vi "Server Single Connection.vi"() -> ()   [LabVIEW 2013]
doc: "This WebSockets API example VI acts as a server for an incoming websockets connection. Receives/sends string data to the connected client."
uses:
  WebSockets/WebSocket Server/WebSocket Server.lvclass
  WebSockets/WebSocket/WebSocket.lvclass/WebSocket.ctl
  WebSockets/WebSocket Server/WebSocket Server.lvclass/WebSocket Server.ctl
  WebSockets/WebSocket/Read Return Headers.vi
  WebSockets/WebSocket Server/Read Request URI.vi
  Sockets/VISA TCP Socket/VISA TCP.lvclass
panel:
  out "Request URI":string
  out "HTTP Headers":variant
  in  "Stop":bool
  out "Received Data":string
  in  "Send":bool
  in  "Data":string
  # "WebSockets Server Example"
  # "This VI is a simple example of sending/receiving data using WebSockets.\nIt waits for a single incoming WebSockets connection on Port 6123 and\nthen displays incoming string data. Strings can also be sent back to the client.\n\nInstructions for use:\n1) Run this VI\n2) Open the index.html file located in the examples folder or the 'Client Single Connection' example\n3) The index.html will display the status of the connection and once established, data can be sent/received from either this VI or the index.html file."
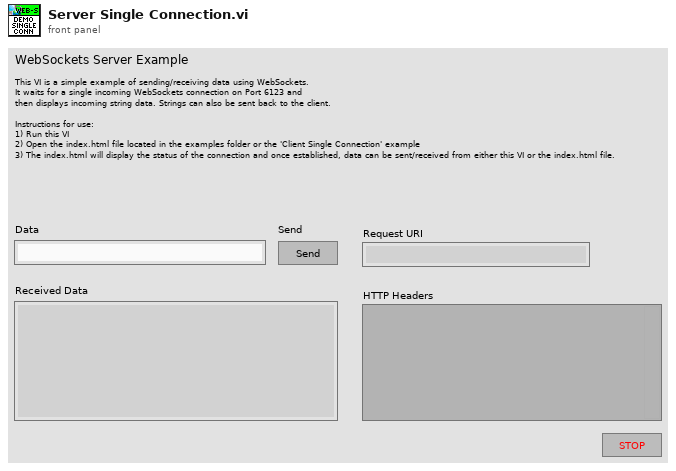
[diagram p1: front panel]
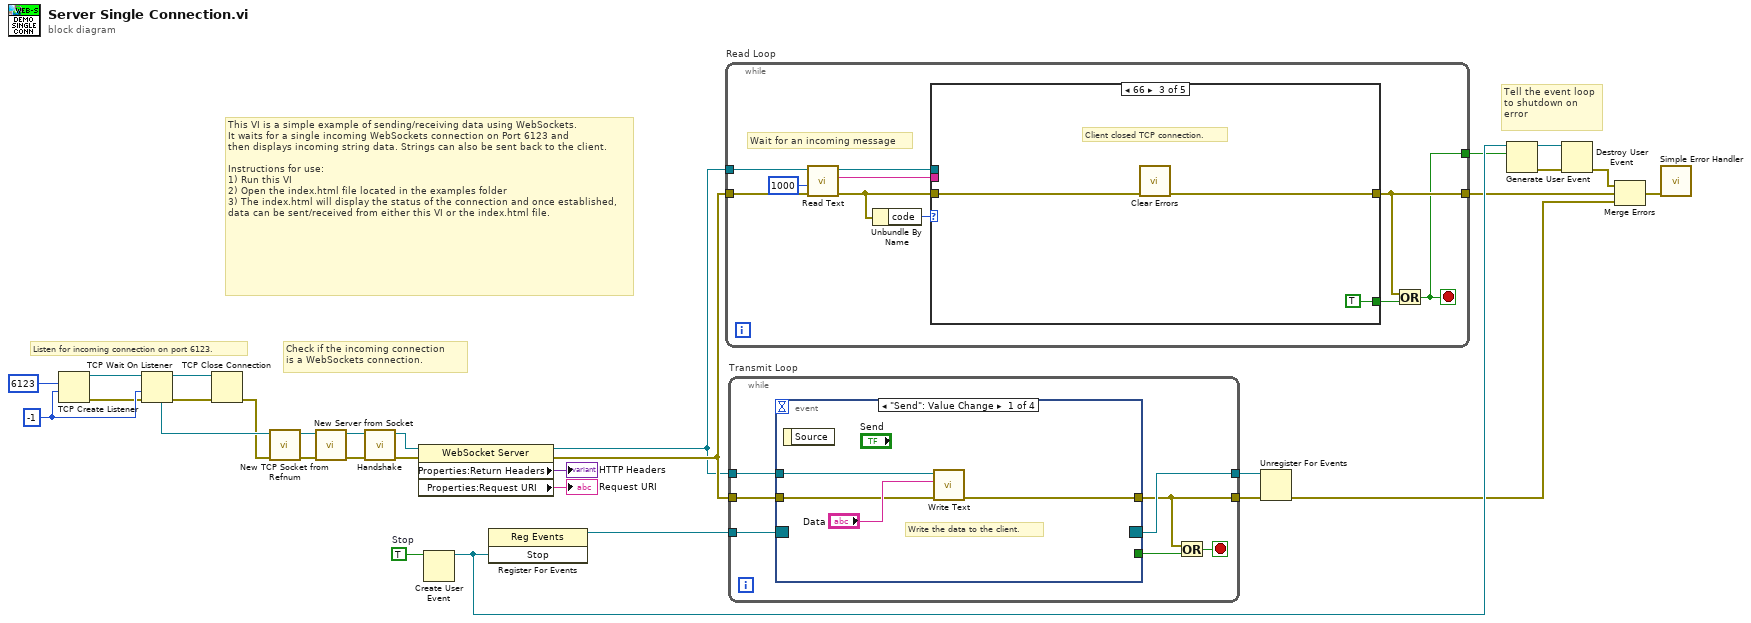
[diagram p0: block diagram]
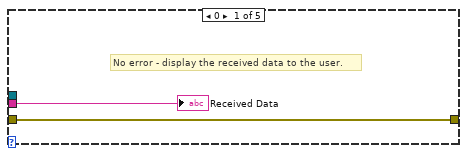
[diagram p2: hidden frame]
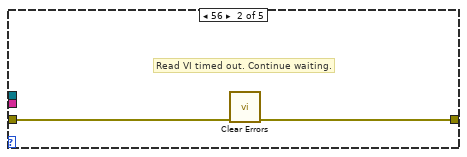
[diagram p3: hidden frame]
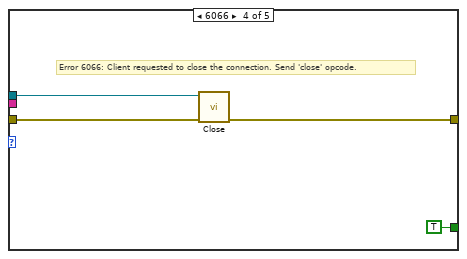
[diagram p4: hidden frame]
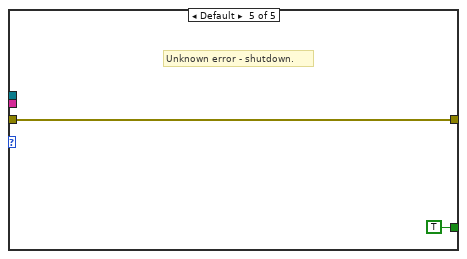
[diagram p5: hidden frame]
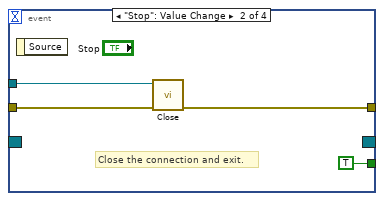
[diagram p6: hidden frame]
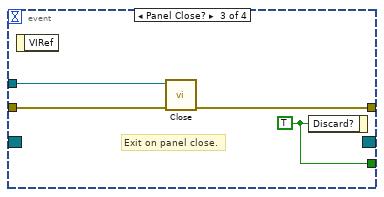
[diagram p7: hidden frame]
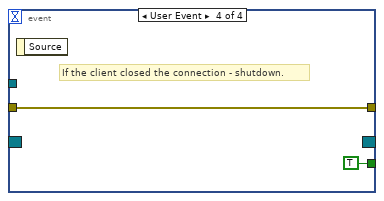
[diagram p8: hidden frame]
diagram:
  w23 = TRUE  # Stop
  w29 = -1 ("timeout ms (25000)")
  # "Tell the event loop to shutdown on error"
  # "This VI is a simple example of sending/receiving data using WebSockets.\nIt waits for a single incoming WebSockets connection on Port 6123 and\nthen displays incoming string data. Strings can also be sent back to the client.\n\nInstructions for use:\n1) Run this VI\n2) Open the index.html file located in the examples folder\n3) The index.html will display the status of the connection and once established, data can be sent/received from either this VI or the index.html file."
  # "Check if the incoming connection\nis a WebSockets connection."
  # "Listen for incoming connection on port 6123."
  n1 = TCP Create Listener(9:w29, 10:u16 6123 ("port")) -> (0:w27:errorcluster, 3:w28:refnum<k5>)  [unwired: 3 in, 1 out]
  n2 = TCP Wait On Listener(8:w27, 9:w29, 11:w28) -> (0:w25:errorcluster, 3:w26:refnum<k5>, 4:w10:refnum<k5>)  [unwired: 1 in, 2 out]
  n3 = TCP Close Connection(connection ID=w26, error in (no error)=w25) -> (error out=w9:errorcluster)  [unwired: 1 in, 1 out]
  n4 = call "New TCP Socket from Refnum.vi"("error in (no error)"=w9, "TCP Network Connection Refnum"=w10) -> ("error out"=w12:errorcluster, "VISA TCP out"=w11:refnum<class "VISA TCP.lvclass">)  [unwired: 8 in]
  n5 = call "New Server from Socket.vi"("error in (no error)"=w12, "Socket"=w11) -> ("error out"=w6:errorcluster, "WebSocket Server out"=w7:refnum<class "WebSocket Server.lvclass">)  [unwired: 8 in]
  n6 = call-dynamic "Handshake.vi"("error in (no error)"=w6, "WebSocket Connection in"=w7) -> ("error out"=w8:errorcluster, "WebSocket Connection out"=w4:refnum<class "WebSocket Server.lvclass">)  [unwired: 8 in]
  n7 = property class="WebSocket Server"(reference=w4, error in=w8) -> (reference out=w3:refnum<class "WebSocket Server.lvclass">, error out=w5:errorcluster, "Properties:Return Headers"=→"HTTP Headers":variant, "Properties:Request URI"=→"Request URI":string)
  n8 = Create User Event(user event datatype=w23) -> (user event=w21:refnum<user-event>)  [unwired: 1 in, 1 out]
  n9 = register-events(w21) -> (reference out=w24:refnum<event-registration>)  [unwired: 2 in, 1 out]
  n10 = while "Read Loop" {
    tunnel: w3 -> [w40]
    tunnel: [w31] -> w20
    tunnel: [w33] -> w14
    tunnel: w5 -> [w34]
    stop <- w31 stop-if-true
    # "Wait for an incoming message"
    n11 = call-dynamic "Read Text.vi"("error in (no error)"=w34, "timeout ms (5000)"=1000 ("timeout ms (25000)"), "WebSocket in"=w40) -> ("error out"=w35:errorcluster, "Data"=w37:string, "WebSocket out"=w36:refnum<class "WebSocket Server.lvclass">)  [unwired: 6 in]
    n12 = Unbundle By Name(w35) -> ("code"=w38:i32)
    n13 = case shown="66" w38 {
      tunnel: w37 -> [w42 _ _ _ _]
      tunnel: [_ _ TRUE TRUE TRUE] -> w32
      tunnel: w36 -> [_ _ _ w51 _]
      tunnel: w35 -> [w41 w44 w46 w49 w52]
      tunnel: [w41 w43 w45 w48 w52] -> w33
      frame 0 {
        # "No error - display the received data to the user."
        "Received Data" <- w42
      }
      frame 56 {
        # "Read VI timed out. Continue waiting."
        n14 = call <vilib>:"Clear Errors.vi"("error in (no error)"=w44) -> ("error out"=w43:errorcluster)  [unwired: 6 in]
      }
      frame 66 {
        # "Client closed TCP connection."
        n15 = call <vilib>:"Clear Errors.vi"("error in (no error)"=w46) -> ("error out"=w45:errorcluster)  [unwired: 6 in]
      }
      frame 6066 {
        # "Error 6066: Client requested to close the connection. Send 'close' opcode."
        n16 = call-dynamic "Close.vi"("error in (no error)"=w49, "WebSocket in"=w51) -> ("error out"=w48:errorcluster)  [unwired: 9 in]
      }
      frame Default {
        # "Unknown error - shutdown."
      }
    }
    n17 = Or(x=w33, y=w32) -> (x .or. y?=w31:bool)
  }
  n18 = while "Transmit Loop" {
    tunnel: w3 -> [w60]
    tunnel: w24 -> [w59]
    tunnel: [w58] -> w22
    tunnel: [w54] -> w15
    tunnel: w5 -> [w57]
    stop <- w55 stop-if-true
    n19 = event shown="[0] \"Send\": Value Change" {
      selector: w59 -> [_ _ _ _]
      dyn-events: [_ _ _ _] -> w58
      timeout: _ -> [_ _ _ _]
      tunnel: w60 -> [w64 w67 w72 _]
      tunnel: [_ TRUE w71 TRUE] -> w56
      tunnel: [w61 w66 w70 w73] -> w54
      tunnel: w57 -> [w62 w65 w69 w73]
      event "Send": Value Change {
        # "Write the data to the client."
        n20 = event-data() -> ()  [unwired: 1 in, 1 out]
        n21 = call-dynamic "Write Text.vi"("error in (no error)"=w62, "String Data"="Data", "WebSocket in"=w64) -> ("error out"=w61:errorcluster)  [unwired: 7 in, 1 out]
      }
      event "Stop": Value Change {
        # "Close the connection and exit."
        n22 = event-data() -> ()  [unwired: 1 in, 1 out]
        n23 = call-dynamic "Close.vi"("error in (no error)"=w65, "WebSocket in"=w67) -> ("error out"=w66:errorcluster)  [unwired: 9 in]
      }
      event Panel Close? {
        w71 = TRUE ("Discard?")
        # "Exit on panel close."
        n24 = event-data() -> ()  [unwired: 1 in, 1 out]
        n25 = call-dynamic "Close.vi"("error in (no error)"=w69, "WebSocket in"=w72) -> ("error out"=w70:errorcluster)  [unwired: 9 in]
        n26 = event-data("Discard?"=w71) -> ()  [unwired: 1 in, 1 out]
      }
      event User Event {
        # "If the client closed the connection - shutdown."
        n27 = event-data() -> ()  [unwired: 1 in, 1 out]
      }
    }
    n28 = Or(x=w54, y=w56) -> (x .or. y?=w55:bool)
  }
  n29 = Unregister For Events(event registration refnum=w22, error in=w15) -> (error out=w13:errorcluster)
  n30 = Generate User Event(user event=w21, event data cluster=w20) -> (user event out=w19:refnum<user-event>, error out=w18:errorcluster)  [unwired: 2 in]
  n31 = Destroy User Event(user event=w19, error in=w18) -> (error out=w17:errorcluster)
  n32 = Merge Errors(w17, w14, w13) -> (w16:errorcluster)
  n33 = call <vilib>:"Simple Error Handler.vi"("error in (no error)"=w16) -> ()  [unwired: 4 in, 5 out]
